vi "is a.vi"(8 "error in (no error)":errorcluster, 11 "Function Generator in":refnum<class "Function Generator.lvclass">) -> (0 "error out":errorcluster, 2 "is a":string, 3 "Function Generator out":refnum<class "Function Generator.lvclass">)   [LabVIEW 2017, in "Hardware.lvlib" / "Function Generator.lvclass"]
uses:
  Function Generator.lvclass
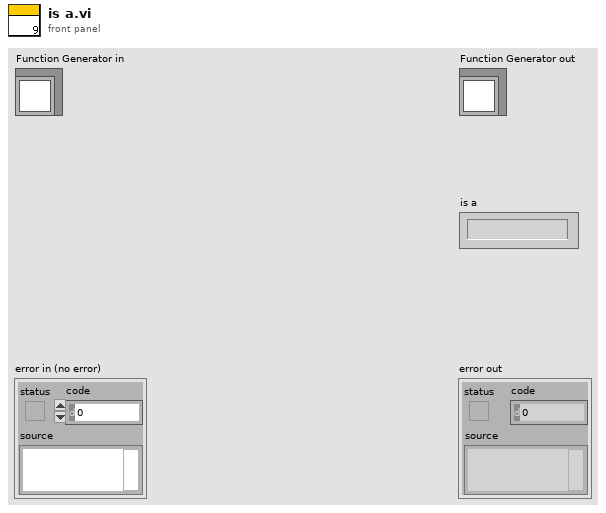
[diagram p1: front panel]
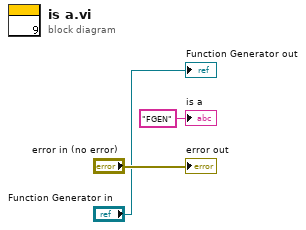
[diagram p0: block diagram]
diagram:
  "error out" <- "error in (no error)"
  "Function Generator out" <- "Function Generator in"
  "is a" <- "FGEN" ("is a")
